vi "Initialize Cameras.vi"(8 "error in":errorcluster, 11 "Gantry in":refnum<class "Gantry Class.lvclass">) -> (0 "error out":errorcluster, 3 "Gantry out":refnum<class "Gantry Class.lvclass">)   [LabVIEW 2011, in "Gantry Class.lvclass"]
uses:
  Gantry Class.lvclass
  Type Definitions/Gantry_Camera.ctl
  <vilib>/userdefined/High Color/IMAQdx.ctl
  Config Manager Class/Type Definitions/Camera Enum.ctl
  <vilib>/vision/driver/NI_Vision_Acquisition_Software.lvlib
  Config Manager Class/Config Manager Class.lvclass
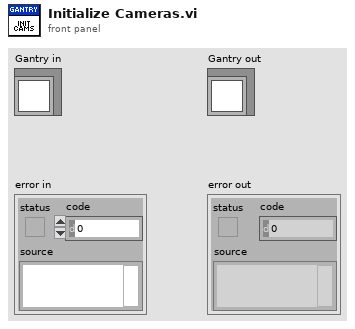
[diagram p1: front panel]
types:
  T1 = typedef "Gantry_Camera.ctl" = cluster{"IMAQ Session":T2, "Group":u32, "Open?":bool, "Interface Name":string, "Field of View":cluster{"x-mm":dbl, "y-mm":dbl}, "Name":T3}
  T2 = typedef "IMAQdx.ctl" = refnum<k21>
  T3 = typedef "Camera Enum.ctl" = enum16{"GANTRY HEAD", "NEEDLE CALIBRATION X", "NEEDLE CALIBRATION Y"}
  T4 = cluster{"Type":u32, "Version":u32, "Flags":u32, "SerialNumberHigh":u32, "SerialNumberLow":u32, "BusType":u32, "InterfaceName":string, "VendorName":string, "ModelName":string, "CameraFileName":string, "CameraAttributeURL":string}
  T5 = cluster{"Type":u32, "Version":u32, "Flags":u32, "SerialNumberHigh":u32, "SerialNumberLow":u32, "BusType":u32, "InterfaceName":string, "VendorName":string, "ModelName":string, "CameraFileName":string, "CameraAttributeURL":string}[]
  T6 = cluster{"Camera Name":T3, "Camera Group":u32, "Camera FOV":cluster{"x":dbl, "y":dbl}}
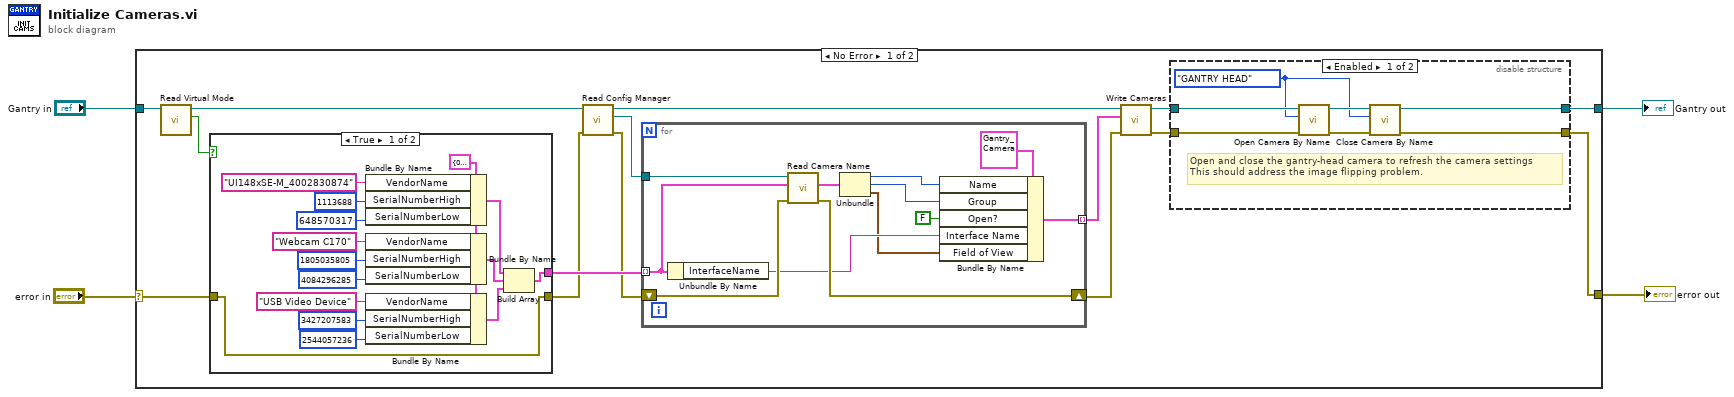
[diagram p0: block diagram]
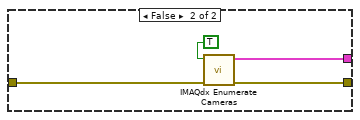
[diagram p3: hidden frame]
diagram:
  n1 = case shown="No Error" "error in" {
    selector: "error in" -> [w17 w61]
    tunnel: [w5 w61] -> w3
    tunnel: [w7 w60] -> w1
    tunnel: "Gantry in" -> [w13 w60]
    frame No Error {
      n2 = call-dynamic "Read Virtual Mode.vi"("Gantry Class in"=w13) -> ("Virtual Mode"=w11:bool, "Gantry Class out"=w12:refnum<class "Gantry Class.lvclass">)  [unwired: 8 in, 1 out]
      n3 = case shown="True" w11 {
        tunnel: [w30 w46] -> w19
        tunnel: w17 -> [w29 w45]
        tunnel: [w29 w44] -> w16
        frame True {
          w34 = T4 {"Type"=0, "Version"=0, "Flags"=0, "SerialNumberHigh"=0, "SerialNumberLow"=0, "BusType"=0, "InterfaceName"="", "VendorName"="", "ModelName"="", "CameraFileName"="", "CameraAttributeURL"=""} ("IMAQdx Data")
          n4 = Bundle By Name(cluster=w34, "VendorName"="UI148xSE-M_4002830874", "SerialNumberHigh"=u32 1113688, "SerialNumberLow"=u32 648570317 ("SerialNumberHigh")) -> (w31:T4)
          n5 = Bundle By Name(cluster=w34, "VendorName"="Webcam C170", "SerialNumberHigh"=u32 1805035805, "SerialNumberLow"=u32 4084296285 ("SerialNumberHigh")) -> (w32:T4)
          n6 = Bundle By Name(cluster=w34, "VendorName"="USB Video Device", "SerialNumberHigh"=u32 3427207583, "SerialNumberLow"=u32 2544057236 ("SerialNumberHigh")) -> (w33:T4)
          n7 = Build Array(w31, w32, w33) -> (w30:T5)
        }
        frame False {
          n8 = call <vilib>:"IMAQdx Enumerate Cameras.vi"("error in"=w45, "Connected Only? (Yes)"=TRUE) -> ("error out"=w44:errorcluster, "Camera Information Array"=w46:T5)  [unwired: 8 in]
        }
      }
      n9 = call-dynamic "Read Config Manager.vi"("error in"=w16, "Gantry in"=w12) -> ("error out"=w15:errorcluster, "Config Manager"=w9:refnum<class "Config Manager Class.lvclass">, "Gantry out"=w10:refnum<class "Gantry Class.lvclass">)  [unwired: 7 in]
      n10 = for {
        tunnel: w19 -> [w58] mode=indexing
        tunnel: [w59] -> w14 mode=indexing
        shift-right: [w55] -> w18
        shift-left: w15 -> [w57]
        tunnel: w9 -> [w52]
        n11 = Unbundle By Name(w58) -> ("InterfaceName"=w54:string)
        n12 = call "Read Camera Name.vi"("error in"=w57, "IMAQdx Data"=w58, "Config Manager in"=w52) -> ("error out"=w55:errorcluster, "Camera Data"=w51:T6)  [unwired: 6 in, 1 out]
        n13 = Unbundle(w51) -> ("Camera Name"=w48:T3, "Camera Group"=w49:u32, "Camera FOV"=w50:cluster{"x":dbl, "y":dbl})
        n14 = Bundle By Name(cluster=T1 {"IMAQ Session"="", "Group"=0, "Open?"=FALSE, "Interface Name"="", "Field of View"={"x-mm"=0.0, "y-mm"=0.0}, "Name"=enum."GANTRY HEAD"} ("Camera"), "Name"=w48, "Group"=w49, "Open?"=FALSE, "Interface Name"=w54, "Field of View"=w50) -> (w59:T1)
      }
      n15 = call-dynamic "Write Cameras.vi"("error in (no error)"=w18, "Cameras"=w14, "Gantry Class in"=w10) -> ("error out"=w6:errorcluster, "Gantry Class out"=w8:refnum<class "Gantry Class.lvclass">)  [unwired: 7 in]
      n16 = disable-structure shown="Enabled" {
        disable-tunnel: w8 -> [w26 w28]
        disable-tunnel: w6 -> [w25 w27]
        disable-tunnel: [w23 w28] -> w7
        disable-tunnel: [w20 w27] -> w5
        frame Enabled {
          w22 = Camera_Enum."GANTRY HEAD" ("Camera Name")
          # "Open and close the gantry-head camera to refresh the camera settings\nThis should address the image flipping problem."
          n17 = call-dynamic "Open Camera By Name.vi"("error in"=w25, "Camera"=w22, "Gantry in"=w26) -> ("error out"=w21:errorcluster, "Gantry out"=w24:refnum<class "Gantry Class.lvclass">)  [unwired: 7 in]
          n18 = call-dynamic "Close Camera By Name.vi"("error in"=w21, "Camera"=w22, "Gantry in"=w24) -> ("error out"=w20:errorcluster, "Gantry out"=w23:refnum<class "Gantry Class.lvclass">)  [unwired: 7 in]
        }
        frame Disabled {
        }
      }
    }
    frame Error {
    }
  }
  "error out" <- w3
  "Gantry out" <- w1
